vi "cw_6_1.vi"() -> ()   [LabVIEW 2022 SP3]
panel:
  out "Count 2":dbl
  out "Count":dbl
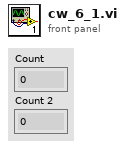
[diagram p1: front panel]
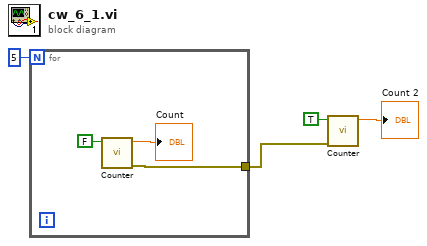
[diagram p0: block diagram]
diagram:
  n1 = for {
    N: 5 -> [_]
    tunnel: [w5] -> w1
    n2 = call "Counter.vi"("Count/Reset"=FALSE) -> ("error constant 2"=w5:errorcluster, "Count"=→"Count":dbl)  [unwired: 9 in]
  }
  n3 = call "Counter.vi"("error constant"=w1, "Count/Reset"=TRUE) -> ("Count"=→"Count 2":dbl)  [unwired: 8 in, 1 out]
